vi "Get Connections - 1Pin 1Conn.vi"(6 "pin type":T1, 7 "instrument type id":string, 8 "error in":errorcluster, 9 "site":i32=-1, 10 "pin or relay name":string, 11 "session reservation in":refnum<class "Session Reservation.lvclass">) -> (0 "error out":errorcluster, 2 "connection":T2, 3 "session reservation out":refnum<class "Session Reservation.lvclass">)   [LabVIEW 2020, in "MeasurementLink VISA.lvlib"]
doc: "Gets the VISA connection information for the given <b>pin type</b>, <b>pin or relay name</b>, and <b>site</b>. If the <b>pin or relay name</b> input is unwired, the connection information for all pins on the given <b>site</b> will be returned. If the <b>site</b> input is unwired, the connection information for the given <b>pin or relay name</b> for all sites will be returned. If both the <b>pin or relay name</b> and <b>site</b> inputs are unwired, the connection information for all pins and on all sites will be returned.\n\nThe <b>pin type</b> input determines what type of pins to get: DUT pins, system pins, or all pins. \n\nIf you have not called <b>Create Sessions.vi</b> prior to calling this VI, the connection information will be returned with the correct information but will have an invalid session.\n\nThis VI returns an error if multiple connections match the inputs. Use <b>Get Connections - 1Pin MConn.vi</b> to get multiple connections from a single pin."
uses:
  MeasurementLink VISA.lvlib
  86b200b6-28cb-4bb1-b3a2-edbec9fb38cc.vi
  MeasurementLink Session Management V1/Session Reservation/Connection.ctl
  MeasurementLink Session Management V1/Session Reservation/Session Reservation.lvclass
  Connection with Session.ctl
  Session Factory/Session Factory.lvclass
  <vilib>/Instr/_visa.llb/VISA Open Access Mode.ctl
  MeasurementLink Session Management V1/Session Reservation/Pin Type.ctl
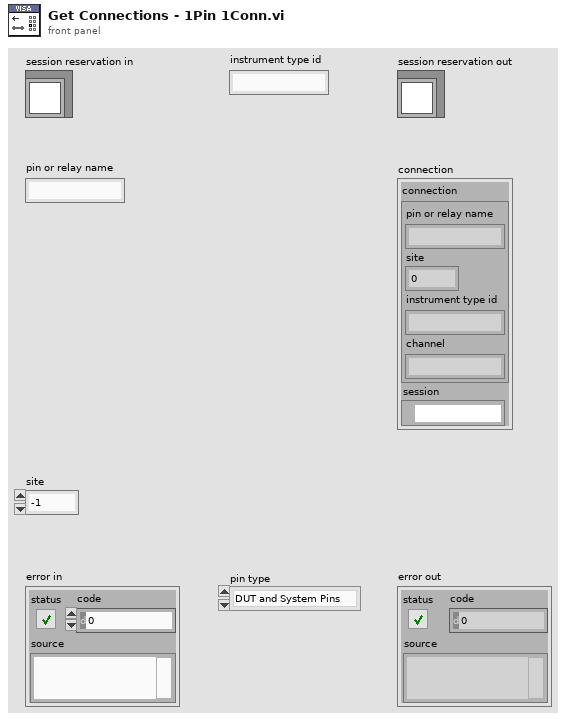
[diagram p1: front panel]
types:
  T1 = typedef "MeasurementLink Session Management V1.lvlib/Session Reservation.lvclass/Pin Type.ctl" = enum16{"DUT and System Pins", "System Pins"}
  T2 = typedef "MeasurementLink VISA.lvlib/Connection with Session.ctl" = cluster{"connection":T3, "session":refnum<visa-resource-name>}
  T3 = typedef "MeasurementLink Session Management V1.lvlib/Session Reservation.lvclass/Connection.ctl" = cluster{"pin or relay name":string, "site":i32, "instrument type id":string, "channel":string}
  T4 = typedef "VISA Open Access Mode.ctl" = u32
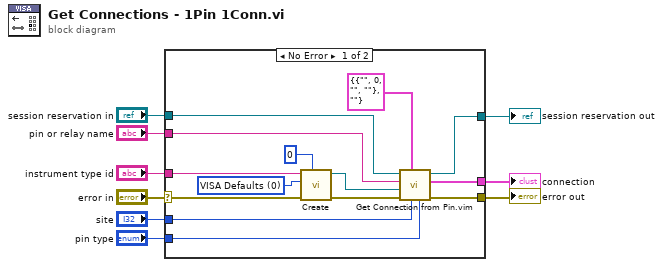
[diagram p0: block diagram]
diagram:
  n1 = case shown="No Error" "error in" {
    selector: "error in" -> [w14 w24]
    tunnel: "session reservation in" -> [w20 w25]
    tunnel: "pin or relay name" -> [w17 _]
    tunnel: [w21 w24] -> w6
    tunnel: [w23 w25] -> w5
    tunnel: [w22 _] -> w4
    tunnel: "site" -> [w19 _]
    tunnel: "pin type" -> [w16 _]
    tunnel: "instrument type id" -> [w15 _]
    frame No Error {
      w10 = T4 0 items=["VISA Defaults"=0, "Exclusive Lock"=1, "Load Configured Settings"=4] ("access mode")
      n2 = call "Create.vi"("visa open timeout"=u32 0, "error in"=w14, "access mode"=w10, "instrument type id"=w15) -> ("error out"=w13:errorcluster, "session factory out"=w12:refnum<class "Session Factory.lvclass">)  [unwired: 6 in]
      n3 = call "Get Connection from Pin.vim"("pin type"=w16, "site"=w19, "connection type"=T2 {"connection"={"pin or relay name"="", "site"=0, "instrument type id"="", "channel"=""}, "session"=""} ("niDCPower connection"), "error in"=w13, "session factory"=w12, "pin or relay name"=w17, "session reservation in"=w20) -> ("error out"=w21:errorcluster, "connection"=w22:T2, "session reservation out"=w23:refnum<class "Session Reservation.lvclass">)  [unwired: 2 in]
    }
    frame Error {
    }
  }
  "error out" <- w6
  "session reservation out" <- w5
  "connection" <- w4
